vi "Stages Messenger_v2.vi"(0 "Stage Notifier Name":string="ProScan3", 2 "Actions":T2, 5 "Setpoint":dbl[](array[numeric]), 7 "Axis":bool[](array[boolean]), 9 "Velocity":dbl, 11 "Misc":variant, 13 "Exit While Busy?":bool) -> (4 "Stage Notifier Name (Dup)":string, 6 "Positions":dbl[](array[numeric]), 8 "Status":T1, 15 "Error":errorcluster)   [LabVIEW 2021]
uses:
  Stages Controls/Stage Actions.ctl
  Stages Controls/Stage Status.ctl
  Stages Controls/Stage Notifier Element.ctl
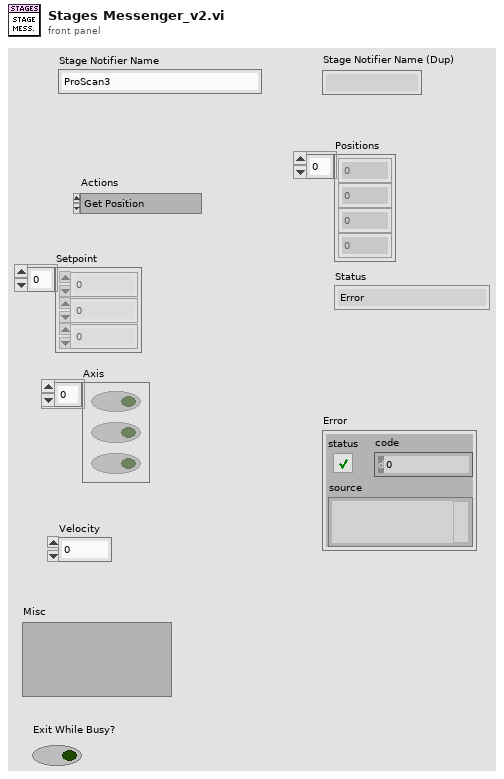
[diagram p1: front panel]
types:
  T1 = typedef "Stage Status.ctl" = enum16{"Error", "Abort", "Busy", "On Target"}
  T2 = typedef "Stage Actions.ctl" = enum16{"Get Position", "SERVO OFF", "SERVO ON", "SERVO ON/OFF", "MVR", "MOVE", "HALT", "ONTARGET", "ERROR", "REFERENCE", "INIT", "VELOCITY", "STATUS", "EXIT", "HOME", "ZEROPOS", "NANOPOS", "ANALOG", "QUIT"}
  T3 = typedef "Stage Notifier Element.ctl" = cluster{"Action":T2, "Axis":bool[], "Setpoint":dbl[], "Velocity":dbl, "Cmd Recvd?":bool, "Position":dbl[], "Status":T1, "Misc":variant, "Servo On?":bool}
  T4 = typedef "Stage Limits.ctl" = cluster{"Notifier":string, "Use Limits":bool, "Limits":dbl[][]}
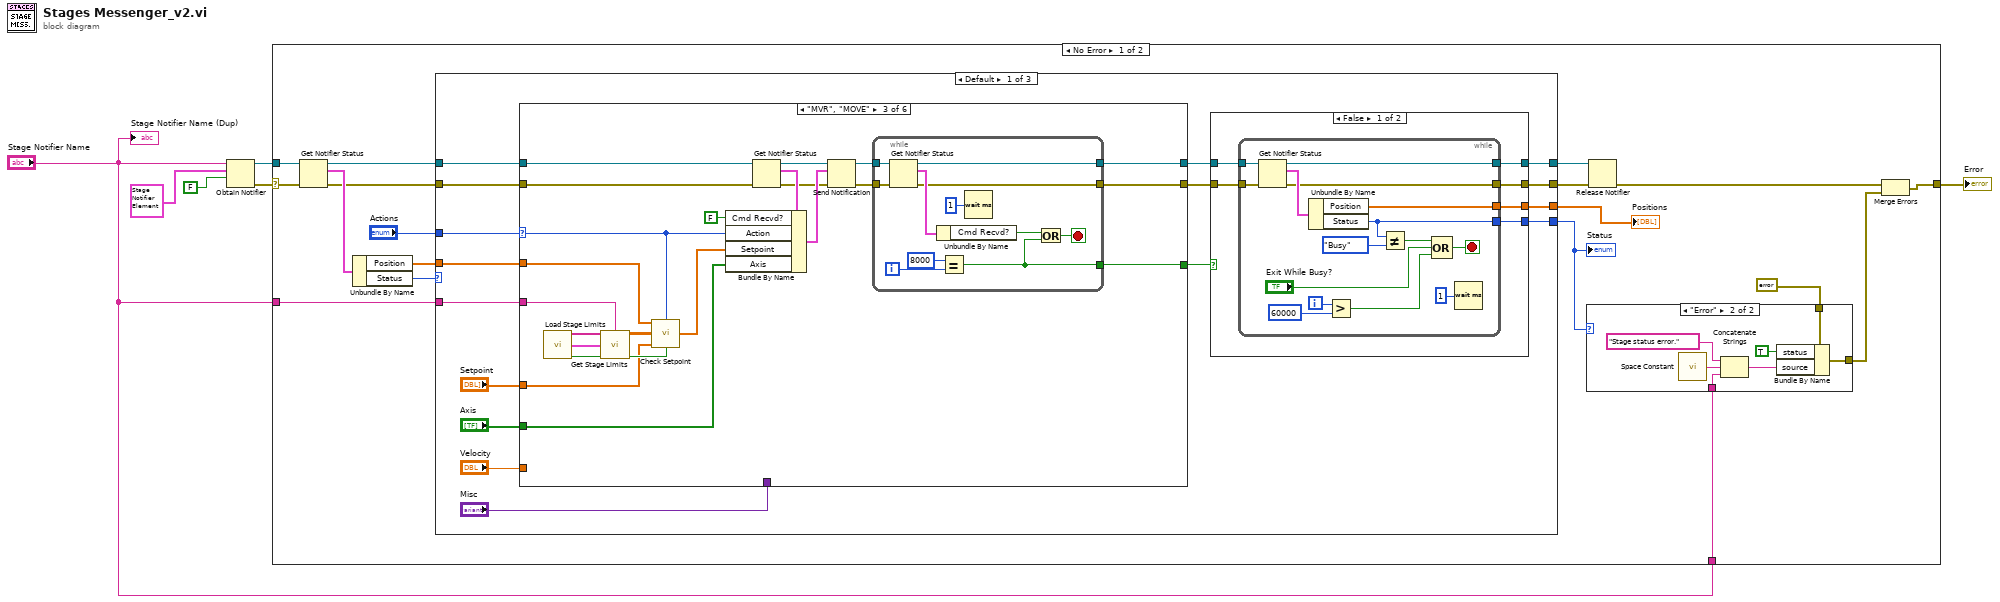
[diagram p0: block diagram]
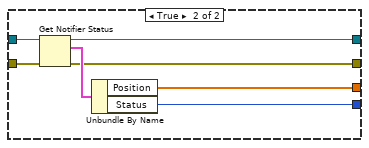
[diagram p3: hidden frame]
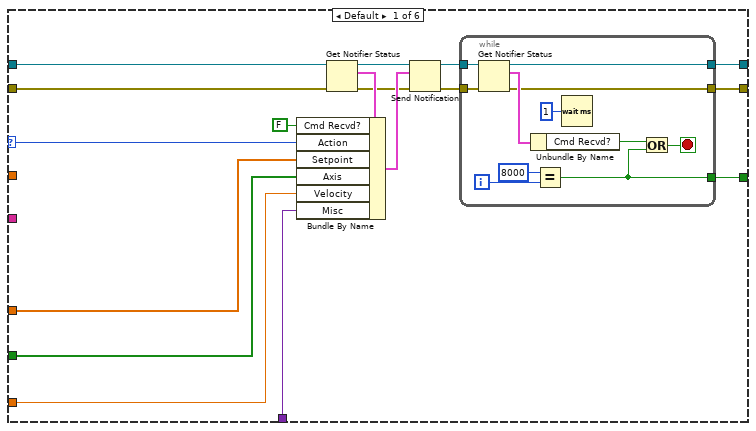
[diagram p4: hidden frame]
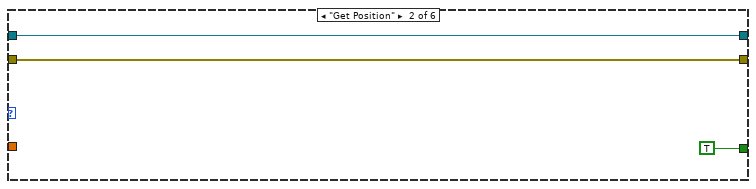
[diagram p5: hidden frame]
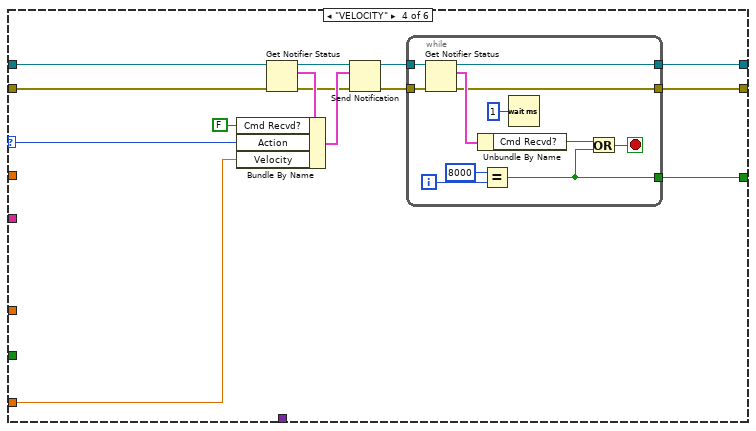
[diagram p6: hidden frame]
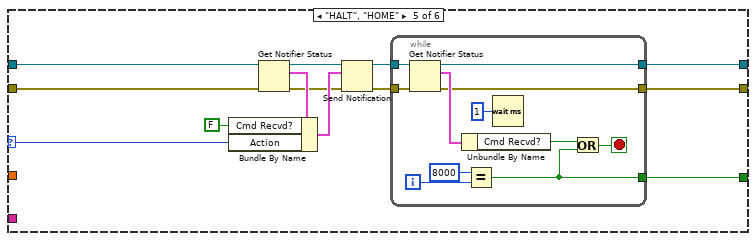
[diagram p7: hidden frame]
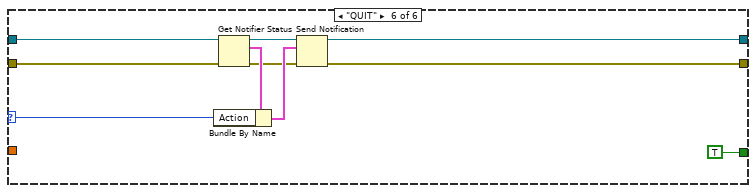
[diagram p8: hidden frame]
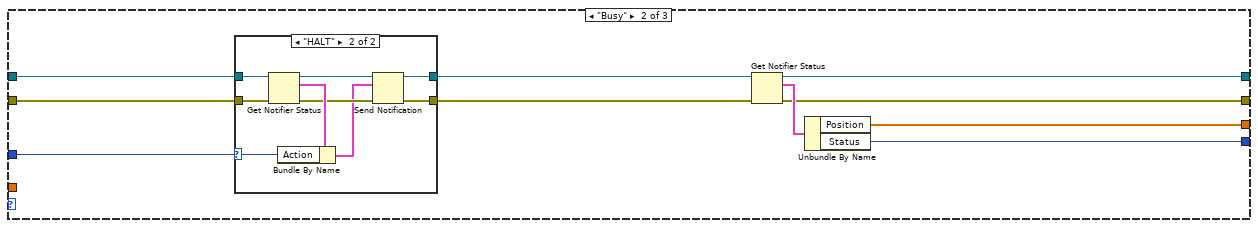
[diagram p9: hidden frame]
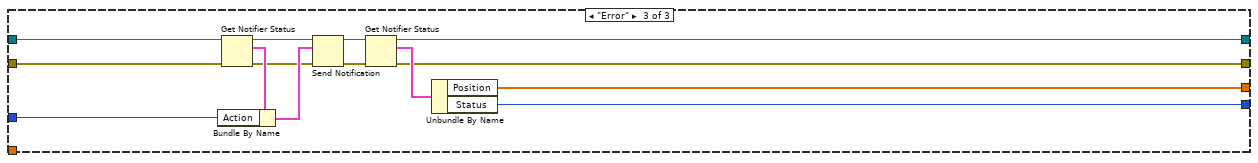
[diagram p11: hidden frame]
diagram:
  n1 = Obtain Notifier(name (unnamed)="Stage Notifier Name", notification data type=T3 {"Action"=enum."Get Position", "Axis"=[], "Setpoint"=[], "Velocity"=0.5, "Cmd Recvd?"=FALSE, "Position"=[], "Status"=enum."Error", "Misc"=variant, "Servo On?"=FALSE} ("Stage Status"), create if not found? (T)=FALSE) -> (notifier out=w3:refnum<notifier>, error out=w4:errorcluster)  [unwired: 1 in, 1 out]
  n2 = case shown="No Error" w4 {
    selector: w4 -> [w18 w236]
    tunnel: w3 -> [w24 _]
    tunnel: "Stage Notifier Name" -> [w13 _]
    tunnel: [w10 w236] -> w2
    tunnel: "Stage Notifier Name" -> [w7 _]
    frame No Error {
      n3 = Get Notifier Status(notifier=w24, error in (no error)=w18) -> (notifier out=w22:refnum<notifier>, current notification=w23:T3, error out=w17:errorcluster)  [unwired: 2 out]
      n4 = Unbundle By Name(w23) -> ("Position"=w8:dbl[], "Status"=w15:T1)
      n5 = case shown="Default" w15 {
        tunnel: w22 -> [w48 w204 w235]
        tunnel: [w41 w209 w229] -> w21
        tunnel: [w40 w208 w228] -> w20
        tunnel: [w39 w207 w227] -> w14
        tunnel: "Actions" -> [w47 w205 w233]
        tunnel: w17 -> [w38 w203 w225]
        tunnel: [w36 w206 w222] -> w16
        tunnel: w8 -> [w34 _ _]
        tunnel: w7 -> [w33 _ _]
        frame Default {
          n6 = case shown="\"MVR\", \"MOVE\"" w47 {
            selector: w47 -> [w89 _ w112 w151 w175 w196]
            tunnel: w48 -> [w90 w107 w127 w152 w176 w199]
            tunnel: [w82 w107 w123 w148 w172 w200] -> w42
            tunnel: "Setpoint" -> [w86 _ w110 _ _ _]
            tunnel: "Axis" -> [w85 _ w124 _ _ _]
            tunnel: "Velocity" -> [w84 _ _ w142 _ _]
            tunnel: "Misc" -> [w83 _ _ _ _ _]
            tunnel: [w81 TRUE w122 w147 w171 TRUE] -> w43
            tunnel: w38 -> [w80 w106 w121 w146 w170 w193]
            tunnel: [w77 w106 w118 w143 w167 w191] -> w37
            tunnel: w34 -> [_ _ w109 _ _ _]
            tunnel: w33 -> [_ _ w117 _ _ _]
            frame Default {
              n7 = Get Notifier Status(notifier=w90, error in (no error)=w80) -> (notifier out=w91:refnum<notifier>, current notification=w92:T3, error out=w79:errorcluster)  [unwired: 2 out]
              n8 = Bundle By Name(cluster=w92, "Cmd Recvd?"=FALSE, "Action"=w89, "Setpoint"=w86, "Axis"=w85, "Velocity"=w84, "Misc"=w83) -> (w93:T3)
              n9 = Send Notification(notification=w93, notifier=w91, error in (no error)=w79) -> (notifier out=w87:refnum<notifier>, error out=w78:errorcluster)
              n10 = while {
                tunnel: w87 -> [w104]
                tunnel: [w101] -> w82
                tunnel: [w97] -> w81
                tunnel: w78 -> [w95]
                tunnel: [w94] -> w77
                i -> [w100]
                stop <- w96 stop-if-true
                n11 = Get Notifier Status(notifier=w104, error in (no error)=w95) -> (notifier out=w101:refnum<notifier>, current notification=w103:T3, error out=w94:errorcluster)  [unwired: 2 out]
                n12 = Unbundle By Name(w103) -> ("Cmd Recvd?"=w98:bool)
                n13 = Equal?(x=8000, y=w100) -> (x = y?=w97:bool)
                n14 = Wait (ms)(milliseconds to wait=u32 1) -> ()  [unwired: 1 out]
                n15 = Or(x=w98, y=w97) -> (x .or. y?=w96:bool)
              }
            }
            frame "Get Position" {
            }
            frame "MVR", "MOVE" {
              n16 = call "Load Stage Limits.vi"() -> ("Notifier Names"=w114:string[], "Stage Limits"=w115:T4[], "Loaded"=w116:bool)  [unwired: 13 in]
              n17 = call "Get Stage Limits.vi"("Notifier Names"=w114, "Notifier Name"=w117, "Stage Limits"=w115, "Limits Loaded?"=w116) -> ("Limits"=w111:dbl[][], "Use Limits?"=w113:bool)  [unwired: 10 in]
              n18 = call "Check Setpoint.vi"("Positions"=w109, "Actions"=w112, "Limits"=w111, "Setpoints"=w110, "Use Limits"=w113) -> ("Setpoints Out"=w108:dbl[])  [unwired: 10 in]
              n19 = Get Notifier Status(notifier=w127, error in (no error)=w121) -> (notifier out=w128:refnum<notifier>, current notification=w129:T3, error out=w120:errorcluster)  [unwired: 2 out]
              n20 = Bundle By Name(cluster=w129, "Cmd Recvd?"=FALSE, "Action"=w112, "Setpoint"=w108, "Axis"=w124) -> (w130:T3)
              n21 = Send Notification(notification=w130, notifier=w128, error in (no error)=w120) -> (notifier out=w125:refnum<notifier>, error out=w119:errorcluster)
              n22 = while {
                tunnel: w125 -> [w141]
                tunnel: [w138] -> w123
                tunnel: [w134] -> w122
                tunnel: w119 -> [w132]
                tunnel: [w131] -> w118
                i -> [w137]
                stop <- w133 stop-if-true
                n23 = Get Notifier Status(notifier=w141, error in (no error)=w132) -> (notifier out=w138:refnum<notifier>, current notification=w140:T3, error out=w131:errorcluster)  [unwired: 2 out]
                n24 = Unbundle By Name(w140) -> ("Cmd Recvd?"=w135:bool)
                n25 = Equal?(x=8000, y=w137) -> (x = y?=w134:bool)
                n26 = Wait (ms)(milliseconds to wait=u32 1) -> ()  [unwired: 1 out]
                n27 = Or(x=w135, y=w134) -> (x .or. y?=w133:bool)
              }
            }
            frame "VELOCITY" {
              n28 = Get Notifier Status(notifier=w152, error in (no error)=w146) -> (notifier out=w153:refnum<notifier>, current notification=w154:T3, error out=w145:errorcluster)  [unwired: 2 out]
              n29 = Bundle By Name(cluster=w154, "Cmd Recvd?"=FALSE, "Action"=w151, "Velocity"=w142) -> (w155:T3)
              n30 = Send Notification(notification=w155, notifier=w153, error in (no error)=w145) -> (notifier out=w149:refnum<notifier>, error out=w144:errorcluster)
              n31 = while {
                tunnel: w149 -> [w166]
                tunnel: [w163] -> w148
                tunnel: [w159] -> w147
                tunnel: w144 -> [w157]
                tunnel: [w156] -> w143
                i -> [w162]
                stop <- w158 stop-if-true
                n32 = Get Notifier Status(notifier=w166, error in (no error)=w157) -> (notifier out=w163:refnum<notifier>, current notification=w165:T3, error out=w156:errorcluster)  [unwired: 2 out]
                n33 = Unbundle By Name(w165) -> ("Cmd Recvd?"=w160:bool)
                n34 = Equal?(x=8000, y=w162) -> (x = y?=w159:bool)
                n35 = Wait (ms)(milliseconds to wait=u32 1) -> ()  [unwired: 1 out]
                n36 = Or(x=w160, y=w159) -> (x .or. y?=w158:bool)
              }
            }
            frame "HALT", "HOME" {
              n37 = Get Notifier Status(notifier=w176, error in (no error)=w170) -> (notifier out=w177:refnum<notifier>, current notification=w178:T3, error out=w169:errorcluster)  [unwired: 2 out]
              n38 = Bundle By Name(cluster=w178, "Cmd Recvd?"=FALSE, "Action"=w175) -> (w179:T3)
              n39 = Send Notification(notification=w179, notifier=w177, error in (no error)=w169) -> (notifier out=w173:refnum<notifier>, error out=w168:errorcluster)
              n40 = while {
                tunnel: w173 -> [w190]
                tunnel: [w187] -> w172
                tunnel: [w183] -> w171
                tunnel: w168 -> [w181]
                tunnel: [w180] -> w167
                i -> [w186]
                stop <- w182 stop-if-true
                n41 = Get Notifier Status(notifier=w190, error in (no error)=w181) -> (notifier out=w187:refnum<notifier>, current notification=w189:T3, error out=w180:errorcluster)  [unwired: 2 out]
                n42 = Unbundle By Name(w189) -> ("Cmd Recvd?"=w184:bool)
                n43 = Equal?(x=8000, y=w186) -> (x = y?=w183:bool)
                n44 = Wait (ms)(milliseconds to wait=u32 1) -> ()  [unwired: 1 out]
                n45 = Or(x=w184, y=w183) -> (x .or. y?=w182:bool)
              }
            }
            frame "QUIT" {
              n46 = Get Notifier Status(notifier=w199, error in (no error)=w193) -> (notifier out=w198:refnum<notifier>, current notification=w197:T3, error out=w192:errorcluster)  [unwired: 2 out]
              n47 = Bundle By Name(cluster=w197, "Action"=w196) -> (w195:T3)
              n48 = Send Notification(notification=w195, notifier=w198, error in (no error)=w192) -> (notifier out=w200:refnum<notifier>, error out=w191:errorcluster)
            }
          }
          n49 = case shown="False" w43 {
            tunnel: w42 -> [w54 w76]
            tunnel: [w53 w75] -> w41
            tunnel: [w52 w74] -> w40
            tunnel: [w51 w72] -> w39
            tunnel: w37 -> [w50 w71]
            tunnel: [w49 w70] -> w36
            frame False {
              n50 = while {
                tunnel: w54 -> [w69]
                tunnel: [w68] -> w53
                tunnel: [w66] -> w52
                tunnel: [w60] -> w51
                tunnel: w50 -> [w56]
                tunnel: [w55] -> w49
                i -> [w62]
                stop <- w57 stop-if-true
                n51 = Get Notifier Status(notifier=w69, error in (no error)=w56) -> (notifier out=w68:refnum<notifier>, current notification=w67:T3, error out=w55:errorcluster)  [unwired: 2 out]
                n52 = Unbundle By Name(w67) -> ("Position"=w66:dbl[], "Status"=w60:T1)
                n53 = Greater?(x=w62, y=60000) -> (0:w58:bool)
                n54 = Not Equal?(x=w60, y=Stage_Status."Busy") -> (x != y?=w63:bool)
                n55 = Compound Arithmetic op=OR(w63, "Exit While Busy?", w58) -> (w57:bool)
                n56 = Wait (ms)(milliseconds to wait=u32 1) -> ()  [unwired: 1 out]
              }
            }
            frame True {
              n57 = Get Notifier Status(notifier=w76, error in (no error)=w71) -> (notifier out=w75:refnum<notifier>, current notification=w73:T3, error out=w70:errorcluster)  [unwired: 2 out]
              n58 = Unbundle By Name(w73) -> ("Position"=w74:dbl[], "Status"=w72:T1)
            }
          }
        }
        frame "Busy" {
          n59 = case shown="\"HALT\"" w205 {
            selector: w205 -> [_ w218]
            tunnel: w204 -> [w212 w221]
            tunnel: w203 -> [w211 w220]
            tunnel: [w212 w215] -> w202
            tunnel: [w211 w214] -> w201
            frame Default {
            }
            frame "HALT" {
              n60 = Get Notifier Status(notifier=w221, error in (no error)=w220) -> (notifier out=w217:refnum<notifier>, current notification=w219:T3, error out=w216:errorcluster)  [unwired: 2 out]
              n61 = Bundle By Name(cluster=w219, "Action"=w218) -> (w213:T3)
              n62 = Send Notification(notification=w213, notifier=w217, error in (no error)=w216) -> (notifier out=w215:refnum<notifier>, error out=w214:errorcluster)
            }
          }
          n63 = Get Notifier Status(notifier=w202, error in (no error)=w201) -> (notifier out=w209:refnum<notifier>, current notification=w210:T3, error out=w206:errorcluster)  [unwired: 2 out]
          n64 = Unbundle By Name(w210) -> ("Position"=w208:dbl[], "Status"=w207:T1)
        }
        frame "Error" {
          n65 = Get Notifier Status(notifier=w235, error in (no error)=w225) -> (notifier out=w232:refnum<notifier>, current notification=w234:T3, error out=w224:errorcluster)  [unwired: 2 out]
          n66 = Bundle By Name(cluster=w234, "Action"=w233) -> (w231:T3)
          n67 = Send Notification(notification=w231, notifier=w232, error in (no error)=w224) -> (notifier out=w230:refnum<notifier>, error out=w223:errorcluster)
          n68 = Get Notifier Status(notifier=w230, error in (no error)=w223) -> (notifier out=w229:refnum<notifier>, current notification=w226:T3, error out=w222:errorcluster)  [unwired: 2 out]
          n69 = Unbundle By Name(w226) -> ("Position"=w228:dbl[], "Status"=w227:T1)
        }
      }
      "Positions" <- w20
      "Status" <- w14
      n70 = case shown="\"Error\"" w14 {
        tunnel: w13 -> [_ w29]
        tunnel: [w25 w27] -> w11
        tunnel: errorcluster {"status"=FALSE, "code"=0, "source"=""} ("Error 2") -> [w25 w26]
        frame Default {
        }
        frame "Error" {
          n71 = call <vilib>:"Space Constant.vi"() -> ("String"=w30:string)
          n72 = Concatenate Strings("Stage status error." ("source"), w30, w29) -> (w28:string)
          n73 = Bundle By Name(cluster=w26, "status"=TRUE, "source"=w28) -> (w27:errorcluster)
        }
      }
      n74 = Release Notifier(notifier=w21, error in (no error)=w16) -> (error out=w12:errorcluster)  [unwired: 1 in, 2 out]
      n75 = Merge Errors(w12, w11) -> (w10:errorcluster)
    }
    frame Error {
    }
  }
  "Error" <- w2
  "Stage Notifier Name (Dup)" <- "Stage Notifier Name"
